vi "ITX Folder to TDMS.vi"(8 "error in (no error)":errorcluster, 11 "LVtoITX in":refnum<class "Data.ITX.lvclass">) -> (0 "error out":errorcluster, 3 "LVtoITX out":refnum<class "Data.ITX.lvclass">)   [LabVIEW 2016, in "Data.TDMS.lvclass"]
uses:
  Data.TDMS.lvclass
  Data.ITX/Data.ITX.lvclass
panel:
  out "Numeric":i32
  in  "Folder Path":path
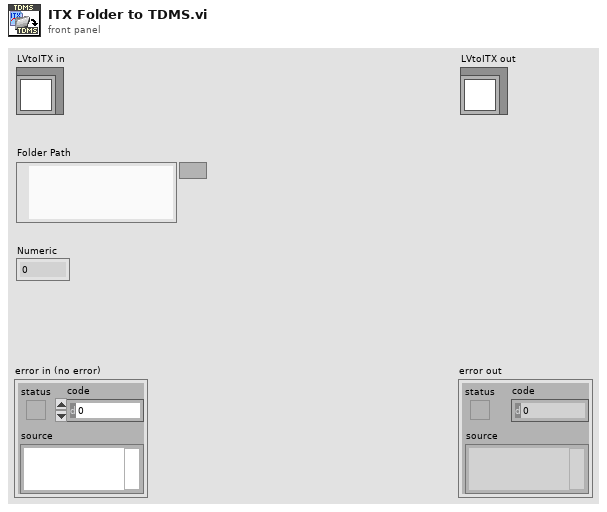
[diagram p1: front panel]
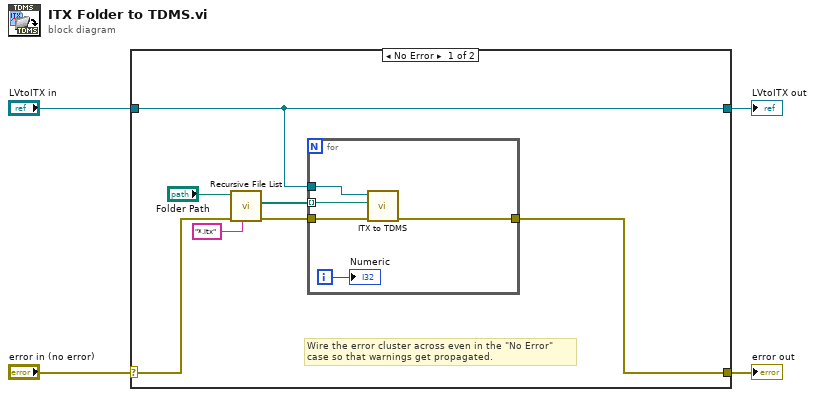
[diagram p0: block diagram]
diagram:
  n1 = case shown="No Error" "error in (no error)" {
    selector: "error in (no error)" -> [w6 w18]
    tunnel: [w5 w18] -> w3
    tunnel: [w8 w17] -> w1
    tunnel: "LVtoITX in" -> [w8 w17]
    frame No Error {
      # "Wire the error cluster across even in the \"No Error\"\ncase so that warnings get propagated."
      n2 = call <vilib>:"Recursive File List.vi"("pattern"="*.itx", "error in (no error)"=w6, "Folder Path"="Folder Path") -> ("error out"=w7:errorcluster, "All Files in Dir"=w9:path[])  [unwired: 4 in, 3 out]
      n3 = for {
        tunnel: w9 -> [w16] mode=indexing
        tunnel: w8 -> [w15]
        tunnel: w7 -> [w14]
        tunnel: [w13] -> w5
        i -> [w12]
        n4 = call "ITX to TDMS.vi"("error in (no error)"=w14, "file (use dialog)"=w16, "LVtoITX in"=w15) -> ("error out"=w13:errorcluster)  [unwired: 7 in, 1 out]
        "Numeric" <- w12
      }
    }
    frame Error {
    }
  }
  "error out" <- w3
  "LVtoITX out" <- w1
